vi "TestMove.vi"() -> ()   [LabVIEW 2017]
uses:
  <vilib>/myRIO/Instrument Drivers/Onboard IO/DIO/typedefs/DIO Reference.ctl
  <vilib>/myRIO/Common/Instrument Driver Framework/Utilities/typedefs/myRIO Generic Hardware Reference.ctl
  <vilib>/myRIO/Common/Instrument Driver Framework/Utilities/typedefs/Hardware Version Enum.ctl
  <vilib>/myRIO/Common/Instrument Driver Framework/Utilities/typedefs/myRIO v1.0 Reference.ctl
  <vilib>/myRIO/Common/Instrument Driver Framework/Utilities/typedefs/Generic FPGA Reference.ctl
  <vilib>/myRIO/Common/Instrument Driver Framework/myRIO v1.0/DIO/typedefs/DIO Channels List.ctl
  <vilib>/myRIO/Common/Instrument Driver Framework/myRIO v1.0/DIO/typedefs/DIO Channels Enum.ctl
  <vilib>/userdefined/High Color/nirio_resource_hc.ctl
  <vilib>/userdefined/High Color/IMAQdx.ctl
  <vilib>/myRIO/Common/Instrument Driver Framework/Utilities/vis/Is FPGA Ref Available.vi
  <vilib>/myRIO/Common/Instrument Driver Framework/myRIO v1.0/DIO/vis/myRIO v1.1 Open DIO.vi
  <vilib>/myRIO/Instrument Drivers/Onboard IO/DIO/vis/Write.vi
  <vilib>/myRIO/Instrument Drivers/Onboard IO/DIO/vis/Read.vi
  <vilib>/myRIO/Common/Instrument Driver Framework/Utilities/vis/Validate Channels.vi
  <vilib>/myRIO/Common/Instrument Driver Framework/myRIO v1.0/DIO/vis/myRIO v1.0 Reserve DIO.vi
  <vilib>/myRIO/Common/Instrument Driver Framework/myRIO v1.0/Resource Manager/vis/myRIO v1.0 Reserve Channel List.vi
  <vilib>/myRIO/Common/Instrument Driver Framework/myRIO v1.0/DIO/vis/myRIO v1.0 Build MUX Configuration DIO.vi
  <vilib>/myRIO/Common/Instrument Driver Framework/myRIO v1.0/Resource Manager/vis/myRIO v1.0 Reserve Channel.vi
  <vilib>/myRIO/Common/Instrument Driver Framework/myRIO v1.0/Resource Manager/vis/myRIO v1.0 Unreserve Channel.vi
  <vilib>/myRIO/Common/Instrument Driver Framework/myRIO v1.0/Resource Manager/vis/myRIO v1.0 Create Configuration List.vi
  <vilib>/myRIO/Common/Instrument Driver Framework/myRIO v1.0/Resource Manager/vis/myRIO v1.0 Build Mutex Name.vi
  <vilib>/Utility/VariantDataType/GetNumericInfo.vi
  <vilib>/Utility/error.llb/Error Cluster From Error Code.vi
  <vilib>/myRIO/Common/Instrument Driver Framework/myRIO v1.0/myRIO v1.1 Open.vi
  <vilib>/myRIO/Common/Instrument Driver Framework/Utilities/vis/IO Manager.vi
  <vilib>/myRIO/Common/Instrument Driver Framework/Utilities/vis/Configuration Manager.vi
  <vilib>/myRIO/Common/Instrument Driver Framework/myRIO v1.0/Resource Manager/vis/myRIO v1.0 Configure IO.vi
  <vilib>/myRIO/Common/Instrument Driver Framework/myRIO v1.0/myRIO v1.0 Close.vi
  <vilib>/myRIO/Common/Instrument Driver Framework/myRIO v1.0/DIO/vis/myRIO v1.0 Write DIO.vi
  <vilib>/myRIO/Common/Instrument Driver Framework/myRIO v1.0/DIO/vis/myRIO v1.0 Read DIO.vi
  Global 5.vi
  <vilib>/myRIO/Express VI/Onboard Devices/LED/LED Express VI.xnode
  <vilib>/myRIO/Instrument Drivers/Onboard IO/DIO/vis/myRIO DIO Open.xnode
  <vilib>/myRIO/Express VI/Onboard Devices/Button/Button Express VI.xnode
  <vilib>/vision/NI_Vision_Development_Module.lvlib
  <vilib>/vision/driver/NI_Vision_Acquisition_Software.lvlib
  <vilib>/myRIO/Instrument Drivers/Onboard IO/DIO/DIO.lvlib
panel:
  out "Data Encode":dbl
  out "Count Encode 2":dbl
  out "x-y":dbl
  out "Back":bool
  out "ROI 2":T1
  out "Im3":T2(plugin-control)
  out "SecondCount":T2(plugin-control)
  out "Number of Objects 3":i32
  out "Less?":bool
  out "Encode Back":dbl
  out "Count Encode":dbl
  out "Status":string
  out "ROI":T1
  out "Count":T2(plugin-control)
  out "Extract":T2(plugin-control)
  out "Particle":T2(plugin-control)
  out "Threshold":T2(plugin-control)
  in  "Settings":T3={"Objects"=0, "Threshold"=128, "Reject Border"=FALSE, "Fill Holes"=FALSE, "Min Object Size"=FALSE, "Min Size"=3, "Max Object Size"=FALSE, "Max Size"=100, "Show Search Area"=FALSE, "Show Center"=TRUE, "Show Bounding Box"=TRUE} {"Objects" items=["Bright Objects", "Dark Objects"]; "Threshold" min=1 max=999999999 step=1; "Max Size" min=1 max=999999999 step=1; "Min Size" min=1 max=999999999 step=1}
  in  "Number of Objects":i32
  out "Number of Objects 2":i32
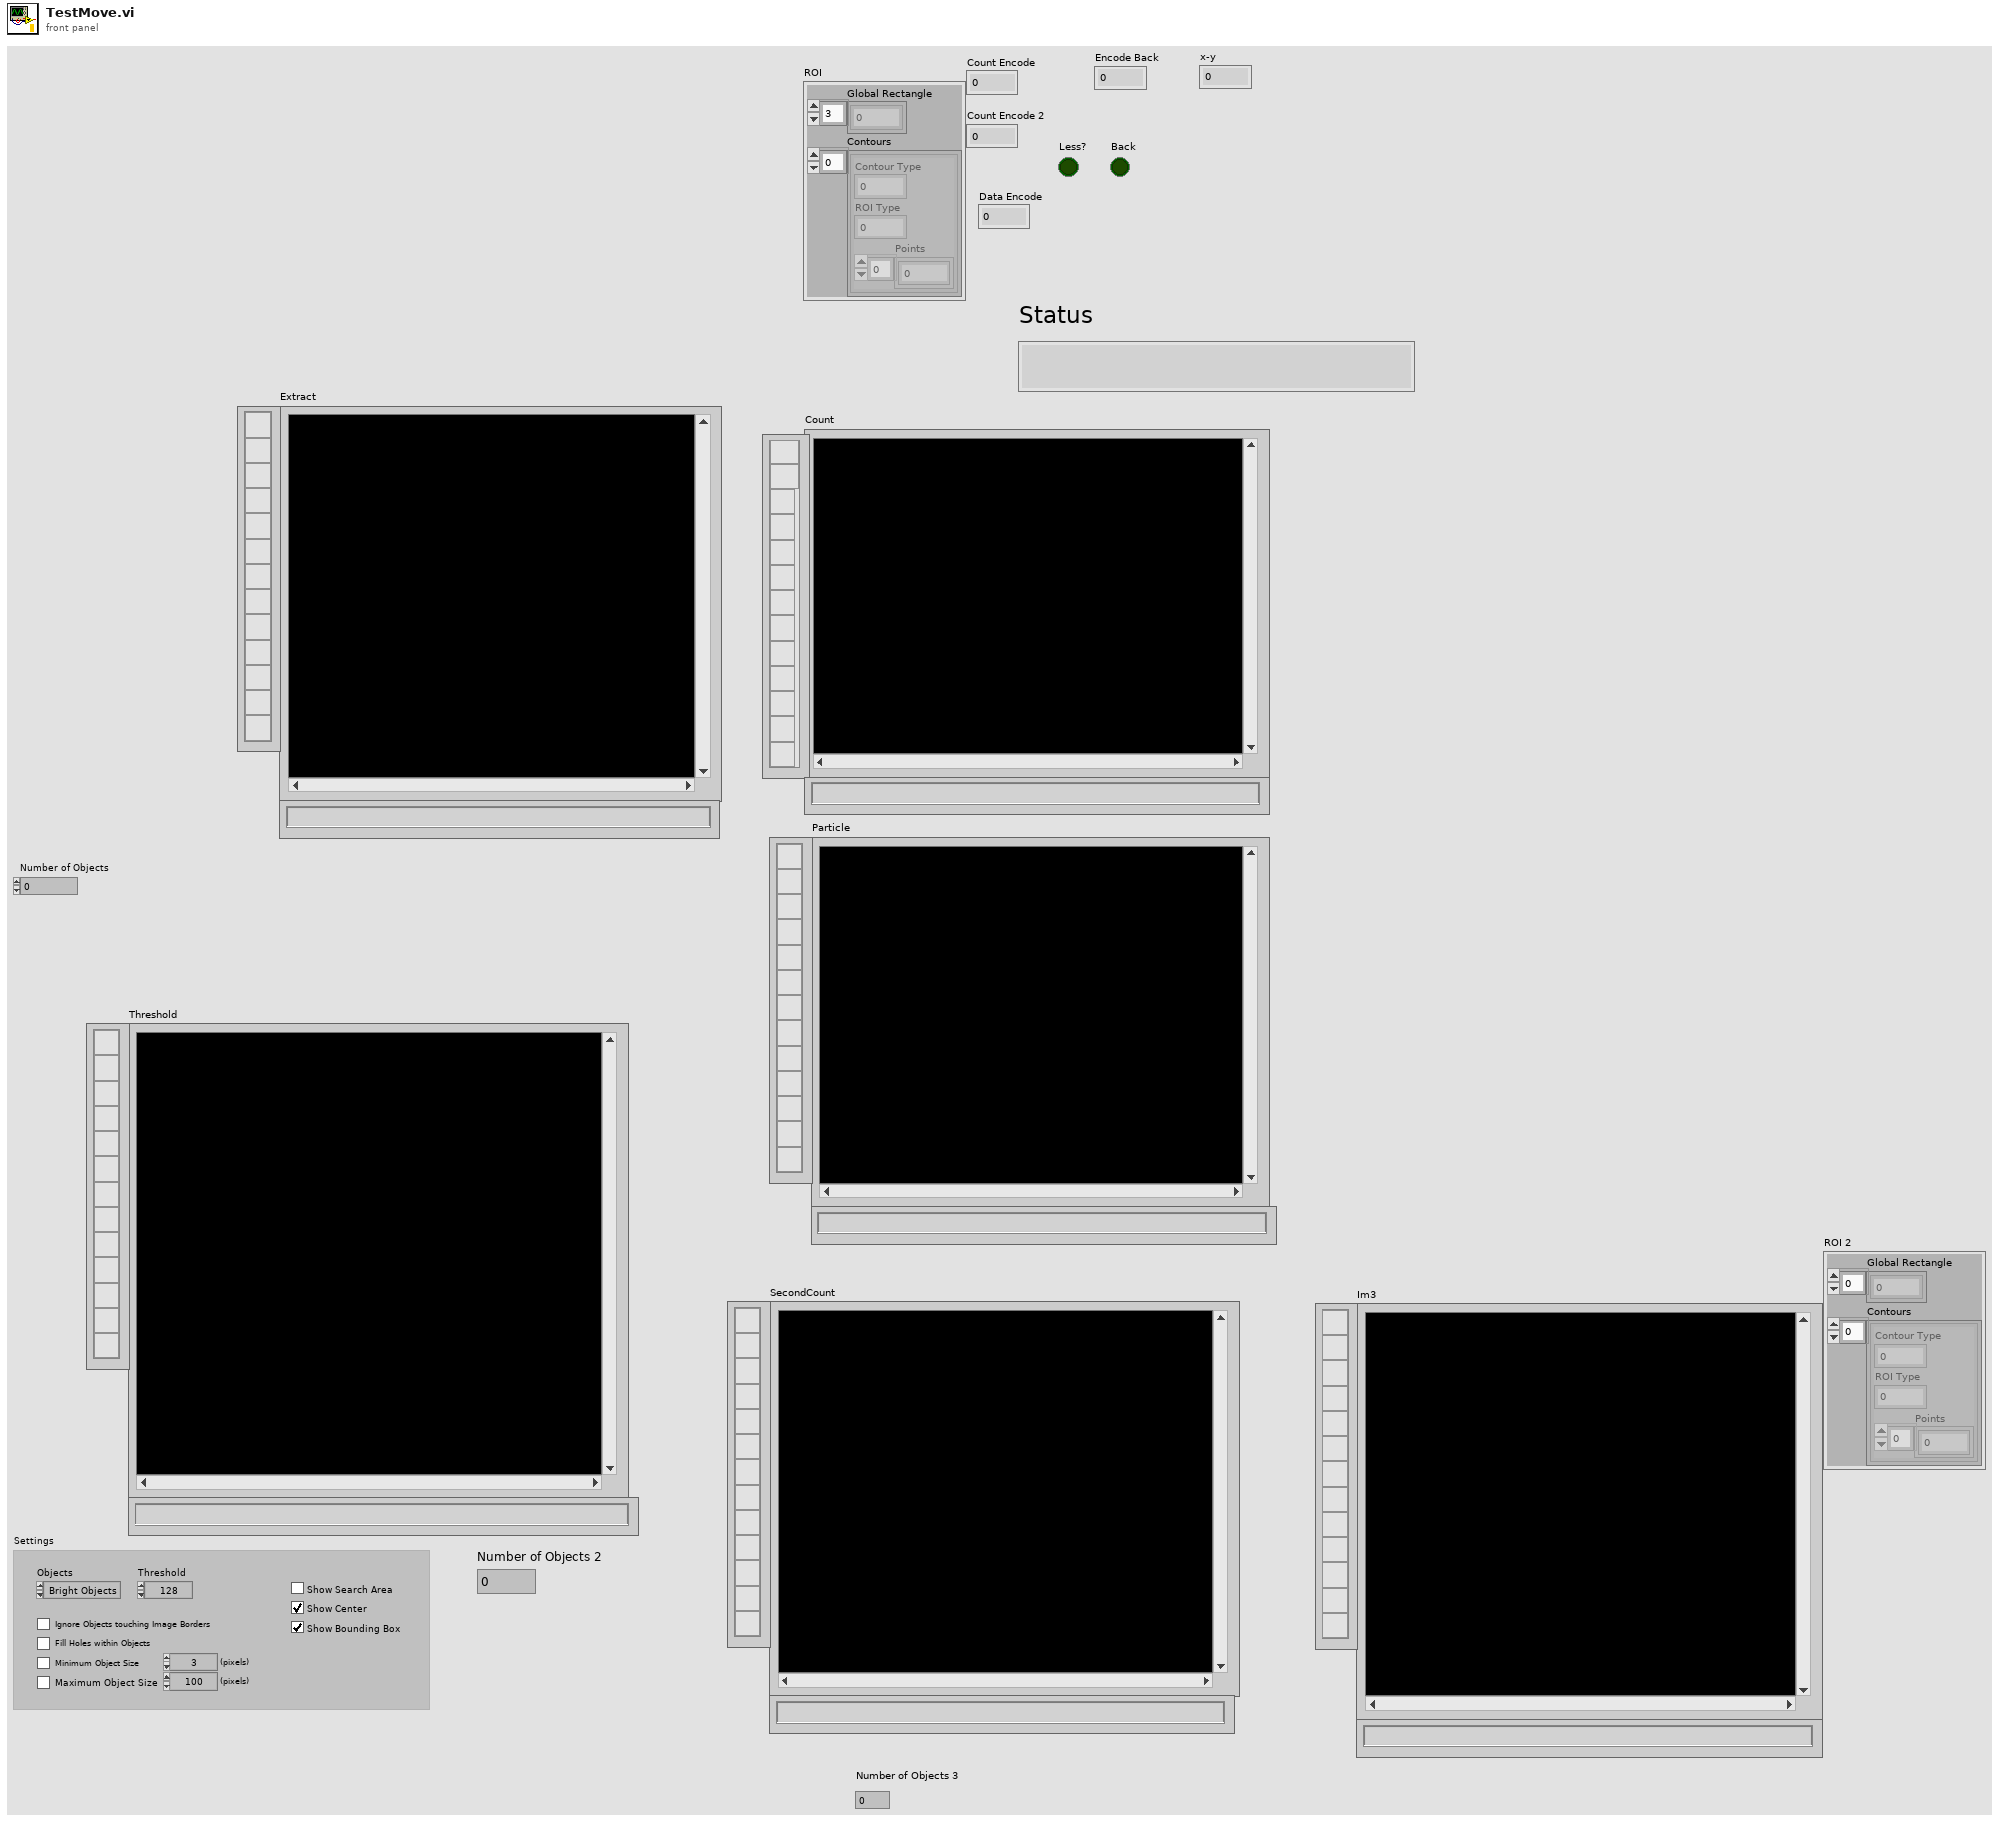
[diagram p1: front panel]
types:
  T1 = cluster{"Global Rectangle":i32[], "Contours":cluster{"Contour Type":u32, "ROI Type":u32, "Points":i32[]}[]}
  T2 = typedef "IMAQ Image.ctl" = refnum<image>
  T3 = cluster{"Objects":u16, "Threshold":i32, "Reject Border":bool, "Fill Holes":bool, "Min Object Size":bool, "Min Size":i32, "Max Object Size":bool, "Max Size":i32, "Show Search Area":bool, "Show Center":bool, "Show Bounding Box":bool}
  T4 = typedef "DIO.lvlib/DIO Reference.ctl" = cluster{"myRIO Reference":T5, "DIO Channels List":T9}
  T5 = typedef "myRIO Generic Hardware Reference.ctl" = cluster{"myRIO Model":T6, "myRIO Hardware Reference":T7}
  T6 = typedef "Hardware Version Enum.ctl" = enum16{"Unknown", "myRIO-1900", "myRIO-1950", "roboRIO", "NI ELVIS RIO CM"}
  T7 = typedef "myRIO v1.0 Reference.ctl" = cluster{"Generic FPGA Reference":T8, "Allow multiple opens":bool}
  T8 = typedef "Generic FPGA Reference.ctl" = refnum<k20>
  T9 = typedef "DIO Channels List.ctl" = T10[]
  T10 = typedef "DIO Channels Enum.ctl" = enum16{"Not Connected", "C/DIO0", "C/DIO1", "C/DIO2", "C/DIO3", "C/DIO4", "C/DIO5", "C/DIO6", "C/DIO7", "A/DIO0", "A/DIO1", "A/DIO2", "A/DIO3", "A/DIO4", "A/DIO5", "A/DIO6", "A/DIO7", "A/DIO8", "A/DIO9", "A/DIO10", "A/DIO11", "A/DIO12", "A/DIO13", "A/DIO14", "A/DIO15", "B/DIO0", "B/DIO1", "B/DIO2", "B/DIO3", "B/DIO4", "B/DIO5", "B/DIO6", "B/DIO7", "B/DIO8", "B/DIO9", "B/DIO10", "B/DIO11", "B/DIO12", "B/DIO13", "B/DIO14", "B/DIO15", "LED0", "LED1", "LED2", "LED3", "Button0", "DIO/DIO0", "DIO/DIO1", "DIO/DIO2", "DIO/DIO3", "DIO/DIO4", "DIO/DIO5", "DIO/DIO6", "DIO/DIO7", "DIO/DIO8", "DIO/DIO9", "SPI/CS0", "SPI/CS1", "SPI/CS2", "SPI/CS3", "LED RADIO (Green)", "LED RADIO (Red)", "LED COMM (Green)", "LED COMM (Red)", "LED MODE (Green)", "LED MODE (Red)"}
  T11 = typedef "nirio_resource_hc.ctl" = tag
  T12 = typedef "IMAQdx.ctl" = refnum<k21>
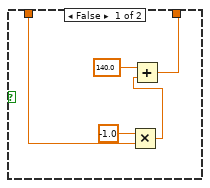
[diagram p2: hidden frame]
diagram:
  n1 = flat-sequence {
    tunnel: [w136] -> w1
    tunnel: [w217] -> w91
    tunnel: [w216] -> w90
    tunnel: [w213] -> w89
    tunnel: w1 -> [w212]
    tunnel: [w263] -> w121
    tunnel: [w262] -> w120
    tunnel: w91 -> [w263]
    tunnel: w90 -> [w262]
    tunnel: w89 -> [w261]
    tunnel: [w260] -> w88
    tunnel: w121 -> [w272]
    tunnel: w120 -> [w271]
    tunnel: [w272] -> w115
    tunnel: [w271] -> w114
    tunnel: w88 -> [w270]
    tunnel: [w269] -> w87
    tunnel: [w282] -> w117
    tunnel: [w281] -> w116
    tunnel: w115 -> [w282]
    tunnel: w114 -> [w281]
    tunnel: w87 -> [w278]
    tunnel: [w276] -> w86
    tunnel: w117 -> [w291]
    tunnel: w116 -> [w290]
    tunnel: [w291] -> w104
    tunnel: [w290] -> w106
    tunnel: w86 -> [w289]
    tunnel: [w288] -> w84
    tunnel: w106 -> [w298]
    tunnel: [w298] -> w105
    tunnel: w104 -> [w297]
    tunnel: [w297] -> w103
    tunnel: [w295] -> w85
    tunnel: w84 -> [w295]
    tunnel: w105 -> [w305]
    tunnel: w103 -> [w304]
    tunnel: [w305] -> w119
    tunnel: [w304] -> w118
    tunnel: w85 -> [w301]
    tunnel: [w299] -> w83
    tunnel: w119 -> [w313]
    tunnel: w118 -> [w314]
    tunnel: [w314] -> w112
    tunnel: [w313] -> w110
    tunnel: w83 -> [w312]
    tunnel: [w311] -> w81
    tunnel: [w321] -> w113
    tunnel: w112 -> [w321]
    tunnel: [w320] -> w111
    tunnel: w110 -> [w320]
    tunnel: [w318] -> w82
    tunnel: w81 -> [w318]
    tunnel: [w324] -> w129
    tunnel: [w326] -> w128
    tunnel: w113 -> [w326]
    tunnel: w111 -> [w324]
    tunnel: w82 -> [w323]
    tunnel: [w322] -> w80
    tunnel: w129 -> [w335]
    tunnel: w128 -> [w336]
    tunnel: [w336] -> w109
    tunnel: [w335] -> w108
    tunnel: w80 -> [w334]
    tunnel: [w333] -> w79
    tunnel: [w344] -> w130
    tunnel: [w345] -> w127
    tunnel: w109 -> [w345]
    tunnel: w108 -> [w344]
    tunnel: w79 -> [w342]
    tunnel: [w340] -> w78
    tunnel: w130 -> [w353]
    tunnel: w127 -> [w354]
    tunnel: w78 -> [w356]
    tunnel: [w355] -> w57
    tunnel: [w354] -> w56
    tunnel: [w353] -> w55
    tunnel: [w361] -> w107
    tunnel: [w362] -> w77
    tunnel: w57 -> [w365]
    tunnel: w56 -> [w364]
    tunnel: w55 -> [w363]
    tunnel: [w360] -> w2
    tunnel: [w424] -> w131
    tunnel: [w425] -> w126
    tunnel: w107 -> [w424]
    tunnel: w77 -> [w422]
    tunnel: [w420] -> w76
    tunnel: w2 -> [w425]
    tunnel: w131 -> [w435]
    tunnel: w126 -> [w434]
    tunnel: [w434] -> w102
    tunnel: [w435] -> w101
    tunnel: [w434] -> w100
    tunnel: w76 -> [w433]
    tunnel: [w432] -> w75
    tunnel: w102 -> [_]
    tunnel: w101 -> [w441]
    tunnel: [w441] -> w66
    tunnel: [w440] -> w65
    tunnel: w100 -> [w440]
    tunnel: w75 -> [w439]
    tunnel: [w439] -> w64
    tunnel: w66 -> [w447]
    tunnel: w65 -> [w448]
    tunnel: [w448] -> w95
    tunnel: [w447] -> w93
    tunnel: w64 -> [w445]
    tunnel: [w443] -> w74
    tunnel: w95 -> [w460]
    tunnel: [w460] -> w94
    tunnel: w93 -> [w461]
    tunnel: [w461] -> w92
    tunnel: w74 -> [w459]
    tunnel: [w458] -> w73
    tunnel: w94 -> [w473]
    tunnel: [w473] -> w99
    tunnel: w92 -> [w474]
    tunnel: [w474] -> w97
    tunnel: w73 -> [w471]
    tunnel: [w469] -> w72
    tunnel: w99 -> [w493]
    tunnel: [w493] -> w98
    tunnel: w97 -> [w492]
    tunnel: [w492] -> w96
    tunnel: w72 -> [w491]
    tunnel: [w490] -> w71
    tunnel: [w500] -> w125
    tunnel: [w501] -> w132
    tunnel: w98 -> [w501]
    tunnel: w96 -> [w500]
    tunnel: w71 -> [w499]
    tunnel: [w497] -> w70
    tunnel: w125 -> [w512]
    tunnel: [w512] -> w124
    tunnel: w132 -> [w511]
    tunnel: [w511] -> w133
    tunnel: w70 -> [w510]
    tunnel: [w509] -> w69
    tunnel: w124 -> [w520]
    tunnel: w133 -> [w521]
    tunnel: [w520] -> w123
    tunnel: [w521] -> w134
    tunnel: w69 -> [w518]
    tunnel: [w516] -> w68
    tunnel: w123 -> [w530]
    tunnel: w134 -> [w531]
    tunnel: [w531] -> w54
    tunnel: [w530] -> w52
    tunnel: w68 -> [w529]
    tunnel: [w528] -> w50
    tunnel: w54 -> [w537]
    tunnel: [w537] -> w53
    tunnel: w52 -> [w536]
    tunnel: [w536] -> w51
    tunnel: w50 -> [w535]
    tunnel: [w535] -> w49
    tunnel: [w543] -> w122
    tunnel: [w544] -> w135
    tunnel: w53 -> [w544]
    tunnel: w51 -> [w543]
    tunnel: w49 -> [w541]
    tunnel: [w539] -> w67
    tunnel: w122 -> [w549]
    tunnel: w135 -> [w550]
    tunnel: w67 -> [w552]
    tunnel: [w551] -> w46
    tunnel: [w550] -> w47
    tunnel: [w549] -> w48
    tunnel: [w559] -> w63
    tunnel: w48 -> [w559]
    tunnel: [w558] -> w62
    tunnel: w47 -> [w558]
    tunnel: [w557] -> w61
    tunnel: w46 -> [w557]
    tunnel: [w563] -> w60
    tunnel: w63 -> [w563]
    tunnel: [w562] -> w59
    tunnel: w62 -> [w562]
    tunnel: w61 -> [w566]
    tunnel: [w561] -> w58
    tunnel: w60 -> [w572]
    tunnel: w59 -> [w573]
    tunnel: w58 -> [w575]
    tunnel: [w574] -> w45
    tunnel: [w573] -> w44
    tunnel: [w572] -> w43
    tunnel: w45 -> [w582]
    tunnel: w44 -> [w580]
    tunnel: w43 -> [w579]
    tunnel: [w579] -> w42
    tunnel: [w581] -> w41
    tunnel: [w580] -> w39
    tunnel: [w579] -> w38
    tunnel: w42 -> [w596]
    tunnel: w41 -> [w595]
    tunnel: [w594] -> w40
    tunnel: w39 -> [w594]
    tunnel: w38 -> [w593]
    tunnel: [w593] -> w37
    tunnel: [w592] -> w33
    tunnel: w40 -> [w605]
    tunnel: w37 -> [w604]
    tunnel: [w603] -> w36
    tunnel: [w602] -> w35
    tunnel: [w601] -> w34
    tunnel: w33 -> [w600]
    tunnel: w36 -> [w658]
    tunnel: w35 -> [w656]
    tunnel: w34 -> [w655]
    tunnel: [w657] -> w32
    tunnel: [w656] -> w31
    tunnel: [w655] -> w30
    tunnel: w32 -> [w670]
    tunnel: w31 -> [w668]
    tunnel: w30 -> [w669]
    tunnel: [w669] -> w29
    tunnel: [w668] -> w27
    tunnel: [w667] -> w24
    tunnel: w29 -> [w677]
    tunnel: [w677] -> w28
    tunnel: w27 -> [w676]
    tunnel: [w676] -> w26
    tunnel: [w674] -> w25
    tunnel: w24 -> [w674]
    tunnel: w28 -> [w682]
    tunnel: w26 -> [w681]
    tunnel: w25 -> [w684]
    tunnel: [w680] -> w23
    tunnel: [w682] -> w22
    tunnel: [w681] -> w21
    tunnel: w23 -> [w695]
    tunnel: w22 -> [w694]
    tunnel: w21 -> [w693]
    tunnel: [w694] -> w20
    tunnel: [w693] -> w19
    tunnel: [w692] -> w18
    tunnel: w20 -> [w701]
    tunnel: w19 -> [w700]
    tunnel: w18 -> [w706]
    tunnel: [w702] -> w17
    tunnel: [w701] -> w15
    tunnel: [w700] -> w13
    tunnel: w17 -> [w715]
    tunnel: [w714] -> w16
    tunnel: w15 -> [w713]
    tunnel: [w713] -> w14
    tunnel: w13 -> [w712]
    tunnel: [w712] -> w12
    tunnel: w16 -> [w720]
    tunnel: w14 -> [w722]
    tunnel: w12 -> [w721]
    tunnel: [w722] -> w11
    tunnel: [w721] -> w9
    tunnel: [w720] -> w7
    tunnel: w11 -> [w733]
    tunnel: [w733] -> w10
    tunnel: w9 -> [w732]
    tunnel: [w732] -> w8
    tunnel: w7 -> [w731]
    tunnel: [w730] -> w6
    tunnel: w10 -> [w739]
    tunnel: w8 -> [w738]
    tunnel: w6 -> [w741]
    tunnel: [w739] -> w5
    tunnel: [w738] -> w4
    tunnel: [w737] -> w3
    tunnel: w5 -> [w751]
    tunnel: w4 -> [w750]
    tunnel: w3 -> [w749]
    frame #0 {
      n2 = while {
        tunnel: [w137] -> w136
        stop <- w139 stop-if-true
        n3 = xnode "Start"("LED0"=TRUE) -> ("error out"=w138:errorcluster)  [unwired: 1 in]
        n4 = xnode "Button"("error in (no error)"=w138) -> ("Value"=w139:bool, "error out"=w137:errorcluster)
      }
    }
    frame #1 {
      w217 = tag "B/I2C" ("myRIO MXP Port A/B")
      w216 = u8 1 ("Controller ID#  (I2C Address)")
      # "enable"
      n5 = Wait (ms)(milliseconds to wait=u32 1000) -> ()  [unwired: 1 out]
      n6 = local write "Status"("Starting" ("Status")) -> ()
      n7 = xnode "Start 2"("LED0"=FALSE) -> ()  [unwired: 1 in, 1 out]
      n8 = call <vilib>:"TETRIX_Enable_DC_Controller_myRIO.vi"("myRIO MXP Port A/B"=w217, "Controller ID#  (I2C Address)"=w216, "Error/Flow In"=w212) -> ("Error/Flow Out"=w215:errorcluster)  [unwired: 4 in]
      n9 = call <vilib>:"TETRIX_Motor_Invert_myRIO.vi"("myRIO MXP Port A/B"=w217, "Invert State"=TRUE, "Select Channel"="Motor 1", "Controller ID#  (I2C Address)"=w216) -> ()  [unwired: 3 in, 1 out]
      n10 = call <vilib>:"TETRIX_Reset_Encoders_myRIO.vi"("myRIO MXP Port A/B"=w217, "Select Encoder"="Encoders 1 and 2", "Controller ID#  (I2C Address)"=w216, "Error/Flow In"=w215) -> ("Error/Flow Out"=w214:errorcluster)  [unwired: 3 in]
      n11 = call <vilib>:"TETRIX_Stop_Motors_myRIO.vi"("myRIO MXP Port A/B"=w217, "Stop Mode"="Brake", "Select Channel"="Both Motors", "Controller ID#  (I2C Address)"=w216, "Error/Flow In"=w214) -> ("Error/Flow Out"=w213:errorcluster)  [unwired: 2 in]
    }
    frame #2 {
      w265 = 700 ("Motor 2 Encoder Target")
      w267 = i16 200 ("Motor 1 Contant Speed (Degrees per Second)")
      # "fate 1 start position"
      n12 = Wait (ms)(milliseconds to wait=u32 5500) -> ()  [unwired: 1 out]
      n13 = call <vilib>:"TETRIX_Set_Motor_Target(s)_myRIO.vi"("Motor 2 Encoder Target"=w265, "Motor 1 Encoder Target"=w265, "myRIO MXP Port A/B"=w263, "Controller ID#  (I2C Address)"=w262, "Motor 2 Constant Speed (Degrees per Second)"=w267, "Motor 1 Contant Speed (Degrees per Second)"=w267, "Encoder Units"="Degrees", "Error/Flow In"=w261) -> ("Error/Flow Out"=w260:errorcluster)  [unwired: 1 in]
      "Status" <- "Phase 1" ("Status")
    }
    frame #3 {
      n14 = Wait (ms)(milliseconds to wait=u32 500) -> ()  [unwired: 1 out]
      n15 = call <vilib>:"TETRIX_Stop_Motors_myRIO.vi"("myRIO MXP Port A/B"=w272, "Stop Mode"="Brake", "Select Channel"="Both Motors", "Controller ID#  (I2C Address)"=w271, "Error/Flow In"=w270) -> ("Error/Flow Out"=w269:errorcluster)  [unwired: 2 in]
    }
    frame #4 {
      w287 = i16 100 ("Motor 1 Contant Speed (Degrees per Second)")
      # "fate 2 catch ball"
      n16 = Wait (ms)(milliseconds to wait=u32 3000) -> ()  [unwired: 1 out]
      n17 = local write "Status"("Turning" ("Status")) -> ()
      n18 = call <vilib>:"TETRIX_Reset_Encoders_myRIO.vi"("myRIO MXP Port A/B"=w282, "Select Encoder"="Encoders 1 and 2", "Controller ID#  (I2C Address)"=w281, "Error/Flow In"=w278) -> ("Error/Flow Out"=w277:errorcluster)  [unwired: 3 in]
      n19 = call <vilib>:"TETRIX_Set_Motor_Target(s)_myRIO.vi"("Motor 2 Encoder Target"=300 ("Motor 1 Encoder Target"), "Motor 1 Encoder Target"=-290, "myRIO MXP Port A/B"=w282, "Controller ID#  (I2C Address)"=w281, "Motor 2 Constant Speed (Degrees per Second)"=w287, "Motor 1 Contant Speed (Degrees per Second)"=w287, "Encoder Units"="Degrees", "Error/Flow In"=w277) -> ("Error/Flow Out"=w276:errorcluster)  [unwired: 1 in]
    }
    frame #5 {
      n20 = Wait (ms)(milliseconds to wait=u32 500) -> ()  [unwired: 1 out]
      n21 = call <vilib>:"TETRIX_Stop_Motors_myRIO.vi"("myRIO MXP Port A/B"=w291, "Stop Mode"="Brake", "Select Channel"="Both Motors", "Controller ID#  (I2C Address)"=w290, "Error/Flow In"=w289) -> ("Error/Flow Out"=w288:errorcluster)  [unwired: 2 in]
    }
    frame #6 {
      n22 = local write "Status"("Move Gripper" ("Status")) -> ()
      n23 = call "ServoPickup.vi"() -> ()  [unwired: 12 in]
    }
    frame #7 {
      w307 = i16 100 ("Motor 1 Contant Speed (Degrees per Second)")
      n24 = Wait (ms)(milliseconds to wait=u32 5000) -> ()  [unwired: 1 out]
      n25 = local write "Status"("Moving to catch" ("Status")) -> ()
      n26 = call <vilib>:"TETRIX_Reset_Encoders_myRIO.vi"("myRIO MXP Port A/B"=w304, "Select Encoder"="Encoders 1 and 2", "Controller ID#  (I2C Address)"=w305, "Error/Flow In"=w301) -> ("Error/Flow Out"=w300:errorcluster)  [unwired: 3 in]
      n27 = call <vilib>:"TETRIX_Set_Motor_Target(s)_myRIO.vi"("Motor 2 Encoder Target"=420 ("Motor 1 Encoder Target"), "Motor 1 Encoder Target"=420, "myRIO MXP Port A/B"=w304, "Controller ID#  (I2C Address)"=w305, "Motor 2 Constant Speed (Degrees per Second)"=w307, "Motor 1 Contant Speed (Degrees per Second)"=w307, "Encoder Units"="Degrees", "Error/Flow In"=w300) -> ("Error/Flow Out"=w299:errorcluster)  [unwired: 1 in]
    }
    frame #8 {
      n28 = Wait (ms)(milliseconds to wait=u32 500) -> ()  [unwired: 1 out]
      n29 = call <vilib>:"TETRIX_Stop_Motors_myRIO.vi"("myRIO MXP Port A/B"=w314, "Stop Mode"="Brake", "Select Channel"="Both Motors", "Controller ID#  (I2C Address)"=w313, "Error/Flow In"=w312) -> ("Error/Flow Out"=w311:errorcluster)  [unwired: 2 in]
    }
    frame #9 {
      n30 = local write "Status"("Catching" ("Status")) -> ()
      n31 = call "PickBall.vi"() -> ()  [unwired: 12 in]
    }
    frame #10 {
      w329 = i16 100 ("Motor 1 Contant Speed (Degrees per Second)")
      n32 = Wait (ms)(milliseconds to wait=u32 4200) -> ()  [unwired: 1 out]
      n33 = call <vilib>:"TETRIX_Set_Motor_Target(s)_myRIO.vi"("Motor 2 Encoder Target"=390 ("Motor 1 Encoder Target"), "Motor 1 Encoder Target"=390, "myRIO MXP Port A/B"=w326, "Controller ID#  (I2C Address)"=w324, "Motor 2 Constant Speed (Degrees per Second)"=w329, "Motor 1 Contant Speed (Degrees per Second)"=w329, "Encoder Units"="Degrees", "Error/Flow In"=w323) -> ("Error/Flow Out"=w322:errorcluster)  [unwired: 1 in]
      n34 = local write "Status"("Moving to Bowling" ("Status")) -> ()
      n35 = call <vilib>:"TETRIX_Reset_Encoders_myRIO.vi"("myRIO MXP Port A/B"=w326, "Select Encoder"="Encoders 1 and 2", "Controller ID#  (I2C Address)"=w324) -> ()  [unwired: 4 in, 1 out]
    }
    frame #11 {
      # "end fate2"
      n36 = Wait (ms)(milliseconds to wait=u32 500) -> ()  [unwired: 1 out]
      n37 = call <vilib>:"TETRIX_Stop_Motors_myRIO.vi"("myRIO MXP Port A/B"=w336, "Stop Mode"="Brake", "Select Channel"="Both Motors", "Controller ID#  (I2C Address)"=w335, "Error/Flow In"=w334) -> ("Error/Flow Out"=w333:errorcluster)  [unwired: 2 in]
    }
    frame #12 {
      w349 = i16 100 ("Motor 2 Constant Speed (Degrees per Second)")
      # "fate 3  go to shoot ball position"
      n38 = Wait (ms)(milliseconds to wait=u32 3000) -> ()  [unwired: 1 out]
      n39 = local write "Status"("Phase 3 Turning" ("Status")) -> ()
      n40 = call <vilib>:"TETRIX_Reset_Encoders_myRIO.vi"("myRIO MXP Port A/B"=w345, "Select Encoder"="Encoders 1 and 2", "Controller ID#  (I2C Address)"=w344, "Error/Flow In"=w342) -> ("Error/Flow Out"=w341:errorcluster)  [unwired: 3 in]
      n41 = call <vilib>:"TETRIX_Set_Motor_Target(s)_myRIO.vi"("Motor 2 Encoder Target"=300, "Motor 1 Encoder Target"=-295, "myRIO MXP Port A/B"=w345, "Controller ID#  (I2C Address)"=w344, "Motor 2 Constant Speed (Degrees per Second)"=w349, "Motor 1 Contant Speed (Degrees per Second)"=w349, "Encoder Units"="Degrees", "Error/Flow In"=w341) -> ("Error/Flow Out"=w340:errorcluster)  [unwired: 1 in]
    }
    frame #13 {
      n42 = Wait (ms)(milliseconds to wait=u32 500) -> ()  [unwired: 1 out]
      n43 = global write "Global 5.vi" "Count Encode"(50.0 ("Count Encode")) -> ()
      n44 = call <vilib>:"TETRIX_Stop_Motors_myRIO.vi"("myRIO MXP Port A/B"=w354, "Stop Mode"="Brake", "Select Channel"="Both Motors", "Controller ID#  (I2C Address)"=w353, "Error/Flow In"=w356) -> ("Error/Flow Out"=w355:errorcluster)  [unwired: 2 in]
    }
    frame #14 {
      (unwired) "im0" ("Image Name")
      n45 = call "IMAQ Create"("Image Name"="im0") -> ("New Image"=w369:T2)  [unwired: 4 in, 1 out]
      n46 = call "IMAQ Create"("Image Name"="im1") -> ("New Image"=w367:T2)  [unwired: 4 in, 1 out]
      n47 = while {
        tunnel: w369 -> [w397]
        tunnel: w367 -> [w394]
        tunnel: w363 -> [w390]
        tunnel: w365 -> [w378]
        tunnel: w364 -> [w373]
        tunnel: [w376] -> w362
        tunnel: [w374] -> w361
        tunnel: [w371] -> w360
        stop <- w388 stop-if-true
        w398 = u16 1 items=["RGB", "HSL", "HSV", "HSI"] ("Color Mode")
        n48 = flat-sequence {
          tunnel: w390 -> [w402]
          tunnel: w378 -> [w407]
          tunnel: [w405] -> w377
          tunnel: [w402] -> w375
          tunnel: w373 -> [w401]
          tunnel: [w401] -> w372
          tunnel: w377 -> [w416]
          tunnel: [w415] -> w376
          tunnel: w375 -> [w414]
          tunnel: [w414] -> w374
          tunnel: w372 -> [w413]
          tunnel: [w413] -> w371
          frame #0 {
            w404 = 50 ("Motor 1 Encoder Target")
            w410 = i16 100 ("Motor 1 Contant Speed (Degrees per Second)")
            n49 = global read "Global 5.vi" "Count Encode"() -> (w408:dbl)
            n50 = Wait (ms)(milliseconds to wait=u32 500 ("millisecond timer value")) -> ()  [unwired: 1 out]
            n51 = Add(x=50.0, y=w408) -> (x+y=w400:dbl)
            "Count Encode" <- w400
            n52 = call <vilib>:"TETRIX_Reset_Encoders_myRIO.vi"("myRIO MXP Port A/B"=w401, "Select Encoder"="Encoders 1 and 2", "Controller ID#  (I2C Address)"=w402, "Error/Flow In"=w407) -> ("Error/Flow Out"=w406:errorcluster)  [unwired: 3 in]
            n53 = call <vilib>:"TETRIX_Set_Motor_Target(s)_myRIO.vi"("Motor 2 Encoder Target"=w404, "Motor 1 Encoder Target"=w404, "myRIO MXP Port A/B"=w401, "Controller ID#  (I2C Address)"=w402, "Motor 2 Constant Speed (Degrees per Second)"=w410, "Motor 1 Contant Speed (Degrees per Second)"=w410, "Encoder Units"="Degrees", "Error/Flow In"=w406) -> ("Error/Flow Out"=w405:errorcluster)  [unwired: 1 in]
            n54 = global write "Global 5.vi" "Count Encode"(w400) -> ()
          }
          frame #1 {
            n55 = Wait (ms)(milliseconds to wait=u32 500 ("millisecond timer value")) -> ()  [unwired: 1 out]
            n56 = call <vilib>:"TETRIX_Stop_Motors_myRIO.vi"("myRIO MXP Port A/B"=w413, "Stop Mode"="Brake", "Select Channel"="Both Motors", "Controller ID#  (I2C Address)"=w414, "Error/Flow In"=w416) -> ("Error/Flow Out"=w415:errorcluster)  [unwired: 2 in]
          }
        }
        n57 = property on="Count" class="ImageControl"() -> ("ROI"=→"ROI":T1)  [unwired: 2 in, 2 out]
        n58 = call <vilib>:"IMAQdx Snap2.vi"("Image In"=w397, "Session In"=T12 "cam0") -> ("Image Out"=w399:T2)  [unwired: 7 in, 2 out]
        n59 = call "IMAQ ExtractColorPlanes"("Blue or Luma or Val or Inten Plane"=w394, "Color Mode"=w398, "Image Src"=w399) -> ("Blue or Luma or Val or Inten Plane out"=w395:T2)  [unwired: 5 in, 3 out]
        n60 = call "IMAQ Rotate"("Angle (degrees)"=sgl -2.3, "Image Src"=w395) -> ("Image Dst Out"=w384:T2)  [unwired: 8 in, 1 out]
        "Count" <- w384
        n61 = call "IMAQ Extract 2"("Optional Rectangle"=i32[] [327, 228, 351, 263], "Image Src"=w384) -> ("Image Dst Out"=w393:T2)  [unwired: 8 in, 1 out]
        "Extract" <- w393
        "Particle" <- w393
        n62 = global read "Global 5.vi" "Count Encode"() -> (w387:dbl)
        n63 = call "IMAQ Count Objects 2"("Settings"="Settings", "Image"=w393) -> ("Number of Objects"=w381:i32, "Image Out"=→"Threshold":T2)  [unwired: 5 in, 3 out]
        "Number of Objects 2" <- w381
        n64 = Greater?(x=w381, y=2) -> (0:w382:bool)
        n65 = Greater Or Equal?(x=w387, y=840.0) -> (x >= y?=w385:bool)
        n66 = Or(x=w382, y=w385) -> (x .or. y?=w388:bool)
      }
      n67 = local write "Status"("IMAQ Start" ("Status")) -> ()
    }
    frame #15 {
      w430 = i16 100 ("Motor 1 Contant Speed (Degrees per Second)")
      n68 = Wait (ms)(milliseconds to wait=u32 3000) -> ()  [unwired: 1 out]
      n69 = local write "Status"("Turning to shoot" ("Status")) -> ()
      n70 = call <vilib>:"TETRIX_Reset_Encoders_myRIO.vi"("myRIO MXP Port A/B"=w425, "Select Encoder"="Encoders 1 and 2", "Controller ID#  (I2C Address)"=w424, "Error/Flow In"=w422) -> ("Error/Flow Out"=w421:errorcluster)  [unwired: 3 in]
      n71 = call <vilib>:"TETRIX_Set_Motor_Target(s)_myRIO.vi"("Motor 2 Encoder Target"=-285, "Motor 1 Encoder Target"=290, "myRIO MXP Port A/B"=w425, "Controller ID#  (I2C Address)"=w424, "Motor 2 Constant Speed (Degrees per Second)"=w430, "Motor 1 Contant Speed (Degrees per Second)"=w430, "Encoder Units"="Degrees", "Error/Flow In"=w421) -> ("Error/Flow Out"=w420:errorcluster)  [unwired: 1 in]
    }
    frame #16 {
      n72 = Wait (ms)(milliseconds to wait=u32 500) -> ()  [unwired: 1 out]
      n73 = call <vilib>:"TETRIX_Stop_Motors_myRIO.vi"("myRIO MXP Port A/B"=w434, "Stop Mode"="Brake", "Select Channel"="Both Motors", "Controller ID#  (I2C Address)"=w435, "Error/Flow In"=w433) -> ("Error/Flow Out"=w432:errorcluster)  [unwired: 2 in]
    }
    frame #17 {
      # "fate 4 shoot ball"
      n74 = local write "Status"(" Shooting" ("Status")) -> ()
      n75 = call "Shoot.vi"() -> ()  [unwired: 12 in]
    }
    frame #18 {
      w453 = i16 100 ("Motor 1 Contant Speed (Degrees per Second)")
      n76 = Wait (ms)(milliseconds to wait=u32 3000) -> ()  [unwired: 1 out]
      n77 = local write "Status"("Turning to Check" ("Status")) -> ()
      n78 = call <vilib>:"TETRIX_Reset_Encoders_myRIO.vi"("myRIO MXP Port A/B"=w448, "Select Encoder"="Encoders 1 and 2", "Controller ID#  (I2C Address)"=w447, "Error/Flow In"=w445) -> ("Error/Flow Out"=w444:errorcluster)  [unwired: 3 in]
      n79 = call <vilib>:"TETRIX_Set_Motor_Target(s)_myRIO.vi"("Motor 2 Encoder Target"=300, "Motor 1 Encoder Target"=-285, "myRIO MXP Port A/B"=w448, "Controller ID#  (I2C Address)"=w447, "Motor 2 Constant Speed (Degrees per Second)"=w453, "Motor 1 Contant Speed (Degrees per Second)"=w453, "Encoder Units"="Degrees", "Error/Flow In"=w444) -> ("Error/Flow Out"=w443:errorcluster)  [unwired: 1 in]
    }
    frame #19 {
      n80 = Wait (ms)(milliseconds to wait=u32 500) -> ()  [unwired: 1 out]
      n81 = local write "Data Encode"(0.0 ("Data Encode")) -> ()
      n82 = local write "Less?"(FALSE ("Less?")) -> ()
      n83 = local write "Encode Back"(0.0 ("Encode Back")) -> ()
      n84 = call <vilib>:"TETRIX_Stop_Motors_myRIO.vi"("myRIO MXP Port A/B"=w460, "Stop Mode"="Brake", "Select Channel"="Both Motors", "Controller ID#  (I2C Address)"=w461, "Error/Flow In"=w459) -> ("Error/Flow Out"=w458:errorcluster)  [unwired: 2 in]
    }
    frame #20 {
      w477 = i16 100 ("Motor 1 Contant Speed (Degrees per Second)")
      n85 = global read "Global 5.vi" "Count Encode"() -> (w466:dbl)
      "Data Encode" <- w466
      n86 = Wait (ms)(milliseconds to wait=u32 5000) -> ()  [unwired: 1 out]
      n87 = local write "Status"("Backwarding" ("Status")) -> ()
      n88 = call <vilib>:"TETRIX_Reset_Encoders_myRIO.vi"("myRIO MXP Port A/B"=w473, "Select Encoder"="Encoders 1 and 2", "Controller ID#  (I2C Address)"=w474, "Error/Flow In"=w471) -> ("Error/Flow Out"=w470:errorcluster)  [unwired: 3 in]
      n89 = Less Or Equal?(x=w466, y=200.0) -> (x <= y?=w468:bool)
      n90 = case shown="True" w468 {
        tunnel: [w480 w485] -> w465
        tunnel: w466 -> [w479 w488]
        frame False {
          n91 = Multiply(x=-1.0, y=w479) -> (x*y=w483:dbl)
          n92 = Add(x=140.0, y=w483) -> (x+y=w480:dbl)
        }
        frame True {
          n93 = Multiply(x=w488, y=-1.0) -> (x*y=w486:dbl)
          n94 = Add(x=80.0, y=w486) -> (x+y=w485:dbl)
          "Less?" <- TRUE ("Less?")
        }
      }
      "Encode Back" <- w465
      n95 = call <vilib>:"TETRIX_Set_Motor_Target(s)_myRIO.vi"("Motor 2 Encoder Target"=w465, "Motor 1 Encoder Target"=w465, "myRIO MXP Port A/B"=w473, "Controller ID#  (I2C Address)"=w474, "Motor 2 Constant Speed (Degrees per Second)"=w477, "Motor 1 Contant Speed (Degrees per Second)"=w477, "Encoder Units"="Degrees", "Error/Flow In"=w470) -> ("Error/Flow Out"=w469:errorcluster)  [unwired: 1 in]
    }
    frame #21 {
      n96 = Wait (ms)(milliseconds to wait=u32 500) -> ()  [unwired: 1 out]
      n97 = call <vilib>:"TETRIX_Stop_Motors_myRIO.vi"("myRIO MXP Port A/B"=w493, "Stop Mode"="Brake", "Select Channel"="Both Motors", "Controller ID#  (I2C Address)"=w492, "Error/Flow In"=w491) -> ("Error/Flow Out"=w490:errorcluster)  [unwired: 2 in]
    }
    frame #22 {
      w507 = i16 100 ("Motor 1 Contant Speed (Degrees per Second)")
      # "fate 5 go home"
      n98 = Wait (ms)(milliseconds to wait=u32 3000) -> ()  [unwired: 1 out]
      n99 = call <vilib>:"TETRIX_Reset_Encoders_myRIO.vi"("myRIO MXP Port A/B"=w501, "Select Encoder"="Encoders 1 and 2", "Controller ID#  (I2C Address)"=w500, "Error/Flow In"=w499) -> ("Error/Flow Out"=w498:errorcluster)  [unwired: 3 in]
      n100 = local write "Status"("Turning to rack" ("Status")) -> ()
      n101 = call <vilib>:"TETRIX_Set_Motor_Target(s)_myRIO.vi"("Motor 2 Encoder Target"=-285, "Motor 1 Encoder Target"=290, "Controller ID#  (I2C Address)"=w500, "Motor 2 Constant Speed (Degrees per Second)"=w507, "Motor 1 Contant Speed (Degrees per Second)"=w507, "Encoder Units"="Degrees", "Error/Flow In"=w498) -> ("Error/Flow Out"=w497:errorcluster)  [unwired: 2 in]
    }
    frame #23 {
      n102 = Wait (ms)(milliseconds to wait=u32 500) -> ()  [unwired: 1 out]
      n103 = call <vilib>:"TETRIX_Stop_Motors_myRIO.vi"("myRIO MXP Port A/B"=w511, "Stop Mode"="Brake", "Select Channel"="Both Motors", "Controller ID#  (I2C Address)"=w512, "Error/Flow In"=w510) -> ("Error/Flow Out"=w509:errorcluster)  [unwired: 2 in]
    }
    frame #24 {
      w526 = i16 100 ("Motor 1 Contant Speed (Degrees per Second)")
      n104 = Wait (ms)(milliseconds to wait=u32 5000) -> ()  [unwired: 1 out]
      n105 = local write "Status"("backwarding to rack " ("Status")) -> ()
      n106 = call <vilib>:"TETRIX_Reset_Encoders_myRIO.vi"("myRIO MXP Port A/B"=w521, "Select Encoder"="Encoders 1 and 2", "Controller ID#  (I2C Address)"=w520, "Error/Flow In"=w518) -> ("Error/Flow Out"=w517:errorcluster)  [unwired: 3 in]
      n107 = call <vilib>:"TETRIX_Set_Motor_Target(s)_myRIO.vi"("Motor 2 Encoder Target"=-400 ("Motor 1 Encoder Target"), "Motor 1 Encoder Target"=-400, "myRIO MXP Port A/B"=w521, "Controller ID#  (I2C Address)"=w520, "Motor 2 Constant Speed (Degrees per Second)"=w526, "Motor 1 Contant Speed (Degrees per Second)"=w526, "Encoder Units"="Degrees", "Error/Flow In"=w517) -> ("Error/Flow Out"=w516:errorcluster)  [unwired: 1 in]
    }
    frame #25 {
      n108 = Wait (ms)(milliseconds to wait=u32 500) -> ()  [unwired: 1 out]
      n109 = call <vilib>:"TETRIX_Stop_Motors_myRIO.vi"("myRIO MXP Port A/B"=w531, "Stop Mode"="Brake", "Select Channel"="Both Motors", "Controller ID#  (I2C Address)"=w530, "Error/Flow In"=w529) -> ("Error/Flow Out"=w528:errorcluster)  [unwired: 2 in]
    }
    frame #26 {
      n110 = call "ServoPickup.vi"() -> ()  [unwired: 12 in]
    }
    frame #27 {
      w538 = 65 ("Motor 1 Encoder Target")
      w548 = i16 100 ("Motor 1 Contant Speed (Degrees per Second)")
      n111 = Wait (ms)(milliseconds to wait=u32 5000) -> ()  [unwired: 1 out]
      n112 = local write "Status"("Go to Rack " ("Status")) -> ()
      n113 = call <vilib>:"TETRIX_Reset_Encoders_myRIO.vi"("myRIO MXP Port A/B"=w544, "Select Encoder"="Encoders 1 and 2", "Controller ID#  (I2C Address)"=w543, "Error/Flow In"=w541) -> ("Error/Flow Out"=w540:errorcluster)  [unwired: 3 in]
      n114 = call <vilib>:"TETRIX_Set_Motor_Target(s)_myRIO.vi"("Motor 2 Encoder Target"=w538, "Motor 1 Encoder Target"=w538, "myRIO MXP Port A/B"=w544, "Controller ID#  (I2C Address)"=w543, "Motor 2 Constant Speed (Degrees per Second)"=w548, "Motor 1 Contant Speed (Degrees per Second)"=w548, "Encoder Units"="Degrees", "Error/Flow In"=w540) -> ("Error/Flow Out"=w539:errorcluster)  [unwired: 1 in]
    }
    frame #28 {
      n115 = Wait (ms)(milliseconds to wait=u32 500) -> ()  [unwired: 1 out]
      n116 = call <vilib>:"TETRIX_Stop_Motors_myRIO.vi"("myRIO MXP Port A/B"=w550, "Stop Mode"="Brake", "Select Channel"="Both Motors", "Controller ID#  (I2C Address)"=w549, "Error/Flow In"=w552) -> ("Error/Flow Out"=w551:errorcluster)  [unwired: 2 in]
    }
    frame #29 {
      n117 = call "PickBall.vi"() -> ()  [unwired: 12 in]
      n118 = local write "Status"(" Catching ball" ("Status")) -> ()
    }
    frame #30 {
      w571 = i16 100 ("Motor 1 Contant Speed (Degrees per Second)")
      n119 = Wait (ms)(milliseconds to wait=u32 4500) -> ()  [unwired: 1 out]
      n120 = call <vilib>:"TETRIX_Reset_Encoders_myRIO.vi"("myRIO MXP Port A/B"=w562, "Select Encoder"="Encoders 1 and 2", "Controller ID#  (I2C Address)"=w563, "Error/Flow In"=w566) -> ("Error/Flow Out"=w565:errorcluster)  [unwired: 3 in]
      n121 = local write "Status"("Move to Shoot " ("Status")) -> ()
      n122 = call <vilib>:"TETRIX_Set_Motor_Target(s)_myRIO.vi"("Motor 2 Encoder Target"=290 ("Motor 1 Encoder Target"), "Motor 1 Encoder Target"=290, "myRIO MXP Port A/B"=w562, "Controller ID#  (I2C Address)"=w563, "Motor 2 Constant Speed (Degrees per Second)"=w571, "Motor 1 Contant Speed (Degrees per Second)"=w571, "Encoder Units"="Degrees", "Error/Flow In"=w565) -> ("Error/Flow Out"=w561:errorcluster)  [unwired: 1 in]
    }
    frame #31 {
      n123 = call <vilib>:"TETRIX_Stop_Motors_myRIO.vi"("myRIO MXP Port A/B"=w573, "Stop Mode"="Brake", "Select Channel"="Both Motors", "Controller ID#  (I2C Address)"=w572, "Error/Flow In"=w575) -> ("Error/Flow Out"=w574:errorcluster)  [unwired: 2 in]
    }
    frame #32 {
      w583 = i16 100 ("Motor 1 Contant Speed (Degrees per Second)")
      n124 = Wait (ms)(milliseconds to wait=u32 4500) -> ()  [unwired: 1 out]
      n125 = local write "Status"("Turning  " ("Status")) -> ()
      n126 = call <vilib>:"TETRIX_Reset_Encoders_myRIO.vi"("myRIO MXP Port A/B"=w580, "Select Encoder"="Encoders 1 and 2", "Controller ID#  (I2C Address)"=w579, "Error/Flow In"=w582) -> ("Error/Flow Out"=w588:errorcluster)  [unwired: 3 in]
      n127 = call <vilib>:"TETRIX_Set_Motor_Target(s)_myRIO.vi"("Motor 2 Encoder Target"=300 ("Motor 1 Encoder Target"), "Motor 1 Encoder Target"=-295, "myRIO MXP Port A/B"=w580, "Controller ID#  (I2C Address)"=w579, "Motor 2 Constant Speed (Degrees per Second)"=w583, "Motor 1 Contant Speed (Degrees per Second)"=w583, "Encoder Units"="Degrees", "Error/Flow In"=w588) -> ("Error/Flow Out"=w581:errorcluster)  [unwired: 1 in]
    }
    frame #33 {
      n128 = global write "Global 5.vi" "Count Encode"(50.0 ("Count Encode")) -> ()
      n129 = Wait (ms)(milliseconds to wait=u32 500) -> ()  [unwired: 1 out]
      n130 = call <vilib>:"TETRIX_Stop_Motors_myRIO.vi"("myRIO MXP Port A/B"=w594, "Stop Mode"="Brake", "Select Channel"="Both Motors", "Controller ID#  (I2C Address)"=w596, "Error/Flow In"=w595) -> ("Error/Flow Out"=w592:errorcluster)  [unwired: 2 in]
    }
    frame #34 {
      n131 = call "IMAQ Create"("Image Name"="im5") -> ("New Image"=w608:T2)  [unwired: 4 in, 1 out]
      n132 = call "IMAQ Create"("Image Name"="im7") -> ("New Image"=w609:T2)  [unwired: 4 in, 1 out]
      n133 = while {
        tunnel: w609 -> [w634]
        tunnel: w608 -> [w628]
        tunnel: w605 -> [w617]
        tunnel: w604 -> [w616]
        tunnel: [w615] -> w603
        tunnel: [w612] -> w602
        tunnel: [w611] -> w601
        tunnel: w600 -> [w610]
        stop <- w623 stop-if-true
        (unwired) 8 ("Number of Objects")
        w632 = u16 1 items=["RGB", "HSL", "HSV", "HSI"] ("Color Mode")
        n134 = flat-sequence {
          tunnel: [w641] -> w618
          tunnel: w617 -> [w639]
          tunnel: w616 -> [w640]
          tunnel: [w640] -> w614
          tunnel: [w639] -> w613
          tunnel: w610 -> [w637]
          tunnel: w618 -> [w651]
          tunnel: [w650] -> w615
          tunnel: w614 -> [w648]
          tunnel: w613 -> [w649]
          tunnel: [w649] -> w612
          tunnel: [w648] -> w611
          frame #0 {
            w642 = 50 ("Motor 1 Encoder Target")
            w645 = i16 100 ("Motor 1 Contant Speed (Degrees per Second)")
            n135 = global read "Global 5.vi" "Count Encode"() -> (w643:dbl)
            n136 = Wait (ms)(milliseconds to wait=u32 500 ("millisecond timer value")) -> ()  [unwired: 1 out]
            n137 = Add(x=50.0, y=w643) -> (x+y=w635:dbl)
            "Count Encode 2" <- w635
            n138 = call <vilib>:"TETRIX_Reset_Encoders_myRIO.vi"("myRIO MXP Port A/B"=w639, "Select Encoder"="Encoders 1 and 2", "Controller ID#  (I2C Address)"=w640, "Error/Flow In"=w637) -> ("Error/Flow Out"=w638:errorcluster)  [unwired: 3 in]
            n139 = call <vilib>:"TETRIX_Set_Motor_Target(s)_myRIO.vi"("Motor 2 Encoder Target"=w642, "Motor 1 Encoder Target"=w642, "myRIO MXP Port A/B"=w639, "Controller ID#  (I2C Address)"=w640, "Motor 2 Constant Speed (Degrees per Second)"=w645, "Motor 1 Contant Speed (Degrees per Second)"=w645, "Encoder Units"="Degrees", "Error/Flow In"=w638) -> ("Error/Flow Out"=w641:errorcluster)  [unwired: 1 in]
            n140 = global write "Global 5.vi" "Count Encode"(w635) -> ()
          }
          frame #1 {
            n141 = Wait (ms)(milliseconds to wait=u32 500 ("millisecond timer value")) -> ()  [unwired: 1 out]
            n142 = call <vilib>:"TETRIX_Stop_Motors_myRIO.vi"("myRIO MXP Port A/B"=w649, "Stop Mode"="Brake", "Select Channel"="Both Motors", "Controller ID#  (I2C Address)"=w648, "Error/Flow In"=w651) -> ("Error/Flow Out"=w650:errorcluster)  [unwired: 2 in]
          }
        }
        n143 = call <vilib>:"IMAQdx Snap2.vi"("Image In"=w634, "Session In"=T12 "cam0") -> ("Image Out"=w633:T2)  [unwired: 7 in, 2 out]
        n144 = call "IMAQ ExtractColorPlanes"("Blue or Luma or Val or Inten Plane"=w628, "Color Mode"=w632, "Image Src"=w633) -> ("Blue or Luma or Val or Inten Plane out"=w631:T2)  [unwired: 5 in, 3 out]
        n145 = call "IMAQ Rotate"("Angle (degrees)"=sgl -2.5, "Image Src"=w631) -> ("Image Dst Out"=w624:T2)  [unwired: 8 in, 1 out]
        "Im3" <- w624
        n146 = call "IMAQ Extract 2"("Optional Rectangle"=i32[] [327, 228, 351, 263], "Image Src"=w624) -> ("Image Dst Out"=w627:T2)  [unwired: 8 in, 1 out]
        n147 = property on="Im3" class="ImageControl"() -> ("ROI"=→"ROI 2":T1)  [unwired: 2 in, 2 out]
        n148 = call "IMAQ Count Objects 2"("Settings"=T3 {"Objects"=0, "Threshold"=128, "Reject Border"=FALSE, "Fill Holes"=FALSE, "Min Object Size"=FALSE, "Min Size"=3, "Max Object Size"=FALSE, "Max Size"=100, "Show Search Area"=FALSE, "Show Center"=TRUE, "Show Bounding Box"=TRUE}, "Image"=w627) -> ("Number of Objects"=w622:i32, "Image Out"=→"SecondCount":T2)  [unwired: 5 in, 3 out]
        "Number of Objects 3" <- w622
        n149 = Greater Or Equal?(x=w622, y=2) -> (x >= y?=w623:bool)
      }
      n150 = local write "Status"("IMAQ Start " ("Status")) -> ()
    }
    frame #35 {
      w665 = i16 100 ("Motor 1 Contant Speed (Degrees per Second)")
      n151 = Wait (ms)(milliseconds to wait=u32 4500) -> ()  [unwired: 1 out]
      n152 = call <vilib>:"TETRIX_Reset_Encoders_myRIO.vi"("myRIO MXP Port A/B"=w656, "Select Encoder"="Encoders 1 and 2", "Controller ID#  (I2C Address)"=w655, "Error/Flow In"=w658) -> ("Error/Flow Out"=w660:errorcluster)  [unwired: 3 in]
      n153 = call <vilib>:"TETRIX_Set_Motor_Target(s)_myRIO.vi"("Motor 2 Encoder Target"=-285 ("Motor 1 Encoder Target"), "Motor 1 Encoder Target"=300, "myRIO MXP Port A/B"=w656, "Controller ID#  (I2C Address)"=w655, "Motor 2 Constant Speed (Degrees per Second)"=w665, "Motor 1 Contant Speed (Degrees per Second)"=w665, "Encoder Units"="Degrees", "Error/Flow In"=w660) -> ("Error/Flow Out"=w657:errorcluster)  [unwired: 1 in]
    }
    frame #36 {
      n154 = Wait (ms)(milliseconds to wait=u32 500) -> ()  [unwired: 1 out]
      n155 = call <vilib>:"TETRIX_Stop_Motors_myRIO.vi"("myRIO MXP Port A/B"=w668, "Stop Mode"="Brake", "Select Channel"="Both Motors", "Controller ID#  (I2C Address)"=w669, "Error/Flow In"=w670) -> ("Error/Flow Out"=w667:errorcluster)  [unwired: 2 in]
    }
    frame #37 {
      n156 = call "Shoot.vi"() -> ()  [unwired: 12 in]
      n157 = local write "Back"(FALSE ("Back")) -> ()
      n158 = local write "Status"("Shooting " ("Status")) -> ()
    }
    frame #38 {
      w688 = i16 100 ("Motor 1 Contant Speed (Degrees per Second)")
      n159 = call <vilib>:"TETRIX_Reset_Encoders_myRIO.vi"("myRIO MXP Port A/B"=w681, "Select Encoder"="Encoders 1 and 2", "Controller ID#  (I2C Address)"=w682, "Error/Flow In"=w684) -> ("Error/Flow Out"=w683:errorcluster)  [unwired: 3 in]
      n160 = local write "Status"("Back Home " ("Status")) -> ()
      n161 = Wait (ms)(milliseconds to wait=u32 4500) -> ()  [unwired: 1 out]
      n162 = call <vilib>:"TETRIX_Set_Motor_Target(s)_myRIO.vi"("Motor 2 Encoder Target"=285, "Motor 1 Encoder Target"=-300, "myRIO MXP Port A/B"=w681, "Controller ID#  (I2C Address)"=w682, "Motor 2 Constant Speed (Degrees per Second)"=w688, "Motor 1 Contant Speed (Degrees per Second)"=w688, "Encoder Units"="Degrees", "Error/Flow In"=w683) -> ("Error/Flow Out"=w680:errorcluster)  [unwired: 1 in]
      "Back" <- TRUE ("Back")
    }
    frame #39 {
      n163 = Wait (ms)(milliseconds to wait=u32 500) -> ()  [unwired: 1 out]
      n164 = call <vilib>:"TETRIX_Stop_Motors_myRIO.vi"("myRIO MXP Port A/B"=w693, "Stop Mode"="Brake", "Select Channel"="Both Motors", "Controller ID#  (I2C Address)"=w694, "Error/Flow In"=w695) -> ("Error/Flow Out"=w692:errorcluster)  [unwired: 2 in]
    }
    frame #40 {
      w709 = i16 200 ("Motor 1 Contant Speed (Degrees per Second)")
      n165 = call <vilib>:"TETRIX_Reset_Encoders_myRIO.vi"("myRIO MXP Port A/B"=w700, "Select Encoder"="Encoders 1 and 2", "Controller ID#  (I2C Address)"=w701, "Error/Flow In"=w706) -> ("Error/Flow Out"=w710:errorcluster)  [unwired: 3 in]
      n166 = Wait (ms)(milliseconds to wait=u32 5000) -> ()  [unwired: 1 out]
      n167 = global read "Global 5.vi" "Count Encode"() -> (w705:dbl)
      n168 = local write "Status"("Encode to Home " ("Status")) -> ()
      n169 = Subtract(x=840.0, y=w705) -> (x-y=w703:dbl)
      "x-y" <- w703
      n170 = call <vilib>:"TETRIX_Set_Motor_Target(s)_myRIO.vi"("Motor 2 Encoder Target"=w703, "Motor 1 Encoder Target"=w703, "myRIO MXP Port A/B"=w700, "Controller ID#  (I2C Address)"=w701, "Motor 2 Constant Speed (Degrees per Second)"=w709, "Motor 1 Contant Speed (Degrees per Second)"=w709, "Encoder Units"="Degrees", "Error/Flow In"=w710) -> ("Error/Flow Out"=w702:errorcluster)  [unwired: 1 in]
    }
    frame #41 {
      n171 = call <vilib>:"TETRIX_Stop_Motors_myRIO.vi"("myRIO MXP Port A/B"=w712, "Stop Mode"="Brake", "Select Channel"="Both Motors", "Controller ID#  (I2C Address)"=w713, "Error/Flow In"=w715) -> ("Error/Flow Out"=w714:errorcluster)  [unwired: 2 in]
      n172 = Wait (ms)(milliseconds to wait=u32 500) -> ()  [unwired: 1 out]
    }
    frame #42 {
      w727 = i16 100 ("Motor 1 Contant Speed (Degrees per Second)")
      n173 = call <vilib>:"TETRIX_Reset_Encoders_myRIO.vi"("myRIO MXP Port A/B"=w721, "Select Encoder"="Encoders 1 and 2", "Controller ID#  (I2C Address)"=w722, "Error/Flow In"=w720) -> ("Error/Flow Out"=w724:errorcluster)  [unwired: 3 in]
      n174 = local write "Status"("Turning" ("Status")) -> ()
      n175 = Wait (ms)(milliseconds to wait=u32 4500) -> ()  [unwired: 1 out]
      n176 = call <vilib>:"TETRIX_Set_Motor_Target(s)_myRIO.vi"("Motor 2 Encoder Target"=290, "Motor 1 Encoder Target"=-295, "myRIO MXP Port A/B"=w721, "Controller ID#  (I2C Address)"=w722, "Motor 2 Constant Speed (Degrees per Second)"=w727, "Motor 1 Contant Speed (Degrees per Second)"=w727, "Encoder Units"="Degrees", "Error/Flow In"=w724) -> ()  [unwired: 1 in, 1 out]
    }
    frame #43 {
      n177 = call <vilib>:"TETRIX_Stop_Motors_myRIO.vi"("myRIO MXP Port A/B"=w732, "Stop Mode"="Brake", "Select Channel"="Both Motors", "Controller ID#  (I2C Address)"=w733, "Error/Flow In"=w731) -> ("Error/Flow Out"=w730:errorcluster)  [unwired: 2 in]
      n178 = Wait (ms)(milliseconds to wait=u32 500) -> ()  [unwired: 1 out]
    }
    frame #44 {
      w745 = i16 200 ("Motor 1 Contant Speed (Degrees per Second)")
      n179 = call <vilib>:"TETRIX_Reset_Encoders_myRIO.vi"("myRIO MXP Port A/B"=w738, "Select Encoder"="Encoders 1 and 2", "Controller ID#  (I2C Address)"=w739, "Error/Flow In"=w741) -> ("Error/Flow Out"=w740:errorcluster)  [unwired: 3 in]
      n180 = Wait (ms)(milliseconds to wait=u32 8000) -> ()  [unwired: 1 out]
      n181 = call <vilib>:"TETRIX_Set_Motor_Target(s)_myRIO.vi"("Motor 2 Encoder Target"=900, "Motor 1 Encoder Target"=900, "myRIO MXP Port A/B"=w738, "Controller ID#  (I2C Address)"=w739, "Motor 2 Constant Speed (Degrees per Second)"=w745, "Motor 1 Contant Speed (Degrees per Second)"=w745, "Encoder Units"="Degrees", "Error/Flow In"=w740) -> ("Error/Flow Out"=w737:errorcluster)  [unwired: 1 in]
    }
    frame #45 {
      n182 = local write "Status"("Welcome Home" ("Status")) -> ()
      n183 = Wait (ms)(milliseconds to wait=u32 500) -> ()  [unwired: 1 out]
      n184 = call <vilib>:"TETRIX_Stop_Motors_myRIO.vi"("myRIO MXP Port A/B"=w750, "Stop Mode"="Brake", "Select Channel"="Both Motors", "Controller ID#  (I2C Address)"=w751, "Error/Flow In"=w749) -> ()  [unwired: 2 in, 1 out]
    }
  }
